vi "LaucherDemoMicroscope.vi"   [LabVIEW 2020]
uses:
  DemoMicrosope.lvclass
  C:/Program Files/National Instruments/LabVIEW 2020/vi.lib/ActorFramework/Actor/Actor.lvclass
  <vilib>/ActorFramework/Actor/Actor.lvclass
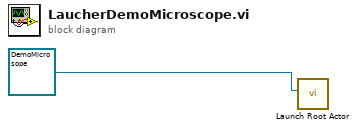
[diagram p0: block diagram]
diagram:
  n1 = call <vilib>:"Launch Root Actor.vi"("Actor"=refnum<class "DemoMicrosope.lvclass"> refnum ("DemoMicrosope.lvlib:DemoMicrosope.lvclass")) -> ()  [unwired: 9 in, 2 out]
